vi "niFpgaButterflyTemp_3Pipe.vi"(0 "x_r":fxp<+/-,16,1>, 1 "mult output type":fxp<+/-,18,2>, 2 "bf bullet type":fxp<+/-,32,16> format="%.21g", 5 "x_i":fxp<+/-,16,1>, 7 "y_r":fxp<+/-,16,1>, 9 "y_i":fxp<+/-,16,1>, 12 "tf_r":fxp<+/-,16,1>, 13 "tf_i":fxp<+/-,16,1>, 14 "first stage":bool) -> (4 "x_out_r":fxp<+/-,16,1>, 6 "x_out_i":fxp<+/-,16,1>, 8 "y_out_r":fxp<+/-,16,1>, 10 "y_out_i":fxp<+/-,16,1>)   [LabVIEW 2017]
uses:
  <vilib>/rvi/FXPMathLib/FxpMul/XNode/nifxpmath_Multiplier.xnode
  <vilib>/rvi/FXPMathLib/sim/FxpSim.dll
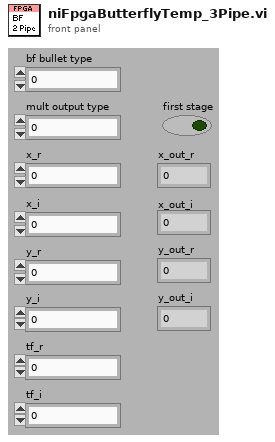
[diagram p1: front panel]
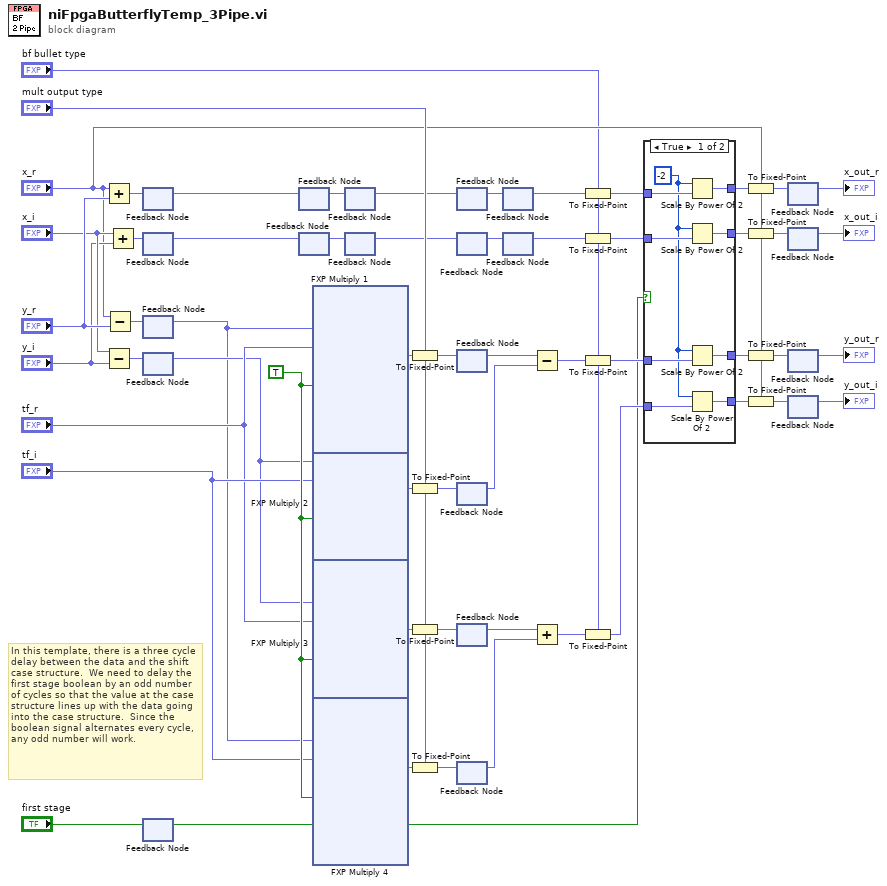
[diagram p0: block diagram]
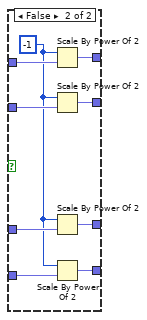
[diagram p2: hidden frame]
diagram:
  w48 = TRUE ("input valid")
  # "In this template, there is a three cycle delay between the data and the shift case structure.  We need to delay the first stage boolean by an odd number of cycles so that the value at the case structure lines up with the data going into the case structure.  Since the boolean signal alternates every cycle, any odd number will work."
  n1 = Add(x="x_r", y="y_r") -> (x+y=w45:fxp<+/-,17,2>)
  n2 = Subtract(x="x_i", y="y_i") -> (x-y=w56:fxp<+/-,17,2>)
  n3 = Subtract(x="x_r", y="y_r") -> (x-y=w57:fxp<+/-,17,2>)
  n4 = Add(x="x_i", y="y_i") -> (x+y=w28:fxp<+/-,17,2>)
  n5 = feedback-in #1(w45) -> ()
  n6 = feedback #1() -> (w32:fxp<+/-,17,2>)  [unwired: 1 out]
  n7 = feedback-in #2(w28) -> ()
  n8 = feedback #2() -> (w30:fxp<+/-,17,2>)  [unwired: 1 out]
  n9 = feedback-in #3(w57) -> ()
  n10 = feedback #3() -> (w26:fxp<+/-,17,2>)  [unwired: 1 out]
  n11 = feedback-in #4(w56) -> ()
  n12 = feedback #4() -> (w27:fxp<+/-,17,2>)  [unwired: 1 out]
  n13 = feedback-in #5("first stage") -> ()
  n14 = feedback #5() -> (w16:bool)  [unwired: 1 out]
  n15 = feedback-in #6(w32) -> ()
  n16 = feedback #6() -> (w31:fxp<+/-,17,2>)  [unwired: 1 out]
  n17 = feedback-in #7(w30) -> ()
  n18 = feedback #7() -> (w29:fxp<+/-,17,2>)  [unwired: 1 out]
  n19 = xnode "FXP Multiply 1"("x"=w26, "y"="tf_r", "input valid"=w48) -> ("x*y"=w17:fxp<+/-,33,3>)  [unwired: 1 in, 2 out]
  n20 = xnode "FXP Multiply 2"("x"=w27, "y"="tf_i", "input valid"=w48) -> ("x*y"=w42:fxp<+/-,33,3>)  [unwired: 1 in, 2 out]
  n21 = xnode "FXP Multiply 3"("x"=w27, "y"="tf_r", "input valid"=w48) -> ("x*y"=w43:fxp<+/-,33,3>)  [unwired: 1 in, 2 out]
  n22 = xnode "FXP Multiply 4"("x"=w26, "y"="tf_i", "input valid"=w48) -> ("x*y"=w44:fxp<+/-,33,3>)  [unwired: 1 in, 2 out]
  n23 = feedback-in #8(w31) -> ()
  n24 = feedback #8() -> (w11:fxp<+/-,17,2>)  [unwired: 1 out]
  n25 = feedback-in #9(w29) -> ()
  n26 = feedback #9() -> (w12:fxp<+/-,17,2>)  [unwired: 1 out]
  n27 = To Fixed-Point(fixed-point type="mult output type", number=w17) -> (fixed-point=w8:fxp<+/-,18,2>)
  n28 = To Fixed-Point(fixed-point type="mult output type", number=w42) -> (fixed-point=w7:fxp<+/-,18,2>)
  n29 = To Fixed-Point(fixed-point type="mult output type", number=w43) -> (fixed-point=w6:fxp<+/-,18,2>)
  n30 = To Fixed-Point(fixed-point type="mult output type", number=w44) -> (fixed-point=w5:fxp<+/-,18,2>)
  n31 = feedback-in #10(w11) -> ()
  n32 = feedback #10() -> (w13:fxp<+/-,17,2>)  [unwired: 1 out]
  n33 = feedback-in #11(w12) -> ()
  n34 = feedback #11() -> (w14:fxp<+/-,17,2>)  [unwired: 1 out]
  n35 = feedback-in #12(w8) -> ()
  n36 = feedback #12() -> (w1:fxp<+/-,18,2>)  [unwired: 1 out]
  n37 = feedback-in #13(w7) -> ()
  n38 = feedback #13() -> (w2:fxp<+/-,18,2>)  [unwired: 1 out]
  n39 = feedback-in #14(w6) -> ()
  n40 = feedback #14() -> (w3:fxp<+/-,18,2>)  [unwired: 1 out]
  n41 = feedback-in #15(w5) -> ()
  n42 = feedback #15() -> (w4:fxp<+/-,18,2>)  [unwired: 1 out]
  n43 = feedback-in #16(w13) -> ()
  n44 = feedback #16() -> (w10:fxp<+/-,17,2>)  [unwired: 1 out]
  n45 = feedback-in #17(w14) -> ()
  n46 = feedback #17() -> (w9:fxp<+/-,17,2>)  [unwired: 1 out]
  n47 = Subtract(x=w1, y=w2) -> (x-y=w37:fxp<+/-,19,3>)
  n48 = Add(x=w3, y=w4) -> (x+y=w39:fxp<+/-,19,3>)
  n49 = To Fixed-Point(fixed-point type="bf bullet type", number=w10) -> (fixed-point=w35:fxp<+/-,32,16>)
  n50 = To Fixed-Point(fixed-point type="bf bullet type", number=w9) -> (fixed-point=w34:fxp<+/-,32,16>)
  n51 = To Fixed-Point(fixed-point type="bf bullet type", number=w37) -> (fixed-point=w36:fxp<+/-,32,16>)
  n52 = To Fixed-Point(fixed-point type="bf bullet type", number=w39) -> (fixed-point=w38:fxp<+/-,32,16>)
  n53 = case shown="True" w16 {
    tunnel: [w66 w75] -> w52
    tunnel: [w65 w74] -> w51
    tunnel: [w64 w73] -> w50
    tunnel: [w63 w72] -> w49
    tunnel: w38 -> [w62 w71]
    tunnel: w36 -> [w61 w70]
    tunnel: w35 -> [w60 w69]
    tunnel: w34 -> [w59 w68]
    frame True {
      w58 = -2 ("n")
      n54 = Scale By Power Of 2(n=w58, x=w60) -> (x*2^n=w66:fxp<+/-,32,16>)
      n55 = Scale By Power Of 2(n=w58, x=w59) -> (x*2^n=w65:fxp<+/-,32,16>)
      n56 = Scale By Power Of 2(n=w58, x=w61) -> (x*2^n=w64:fxp<+/-,32,16>)
      n57 = Scale By Power Of 2(n=w58, x=w62) -> (x*2^n=w63:fxp<+/-,32,16>)
    }
    frame False {
      w67 = -1 ("n")
      n58 = Scale By Power Of 2(n=w67, x=w69) -> (x*2^n=w75:fxp<+/-,32,16>)
      n59 = Scale By Power Of 2(n=w67, x=w68) -> (x*2^n=w74:fxp<+/-,32,16>)
      n60 = Scale By Power Of 2(n=w67, x=w70) -> (x*2^n=w73:fxp<+/-,32,16>)
      n61 = Scale By Power Of 2(n=w67, x=w71) -> (x*2^n=w72:fxp<+/-,32,16>)
    }
  }
  n62 = To Fixed-Point(fixed-point type="x_r", number=w52) -> (fixed-point=w24:fxp<+/-,16,1>)
  n63 = To Fixed-Point(fixed-point type="x_r", number=w51) -> (fixed-point=w25:fxp<+/-,16,1>)
  n64 = To Fixed-Point(fixed-point type="x_r", number=w50) -> (fixed-point=w23:fxp<+/-,16,1>)
  n65 = To Fixed-Point(fixed-point type="x_r", number=w49) -> (fixed-point=w22:fxp<+/-,16,1>)
  n66 = feedback-in #18(w24) -> ()
  n67 = feedback #18() -> (→"x_out_r":fxp<+/-,16,1>)  [unwired: 1 out]
  n68 = feedback-in #19(w25) -> ()
  n69 = feedback #19() -> (→"x_out_i":fxp<+/-,16,1>)  [unwired: 1 out]
  n70 = feedback-in #20(w23) -> ()
  n71 = feedback #20() -> (→"y_out_r":fxp<+/-,16,1>)  [unwired: 1 out]
  n72 = feedback-in #21(w22) -> ()
  n73 = feedback #21() -> (→"y_out_i":fxp<+/-,16,1>)  [unwired: 1 out]
